vi "SQLite Adding Tests.vi"(8 "Error In (no error)":errorcluster) -> (0 "Error Out":errorcluster)   [LabVIEW 2023]
uses:
  <vilib>/addons/_JKI Toolkits/Caraya/classes/Test/Test.lvclass
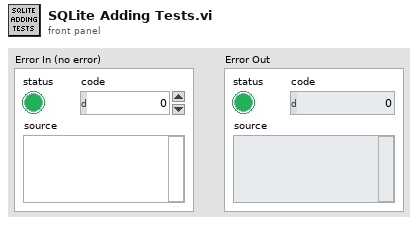
[diagram p1: front panel]
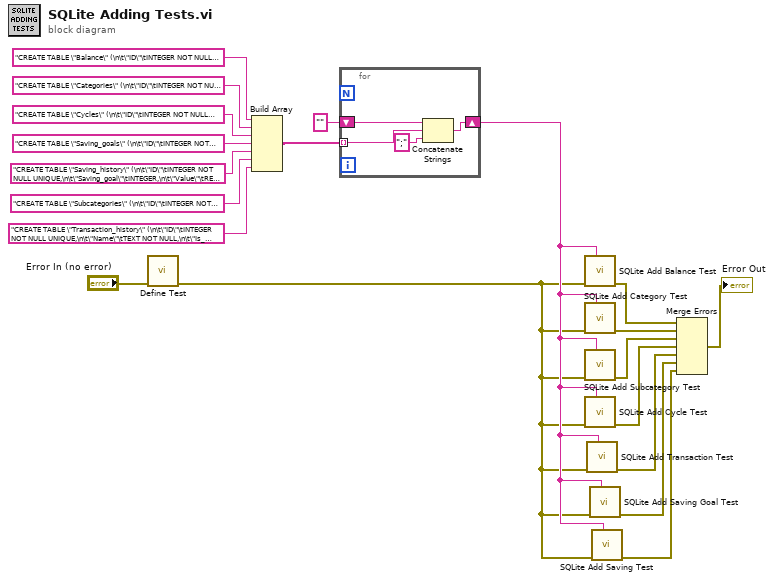
[diagram p0: block diagram]
diagram:
  n1 = call <vilib>:"Define Test.vi"("error in (no error)"="Error In (no error)") -> ("error out"=w2:errorcluster)  [unwired: 9 in, 1 out]
  n2 = Build Array("CREATE TABLE \"Balance\" (\n\t\"ID\"\tINTEGER NOT NULL UNIQUE,\n\t\"Value\"\tREAL NOT NULL,\n\t\"Last_update\"\tREAL NOT NULL,\n\tPRIMARY KEY(\"ID\" AUTOINCREMENT)\n);\nCREATE TRIGGER Balance_single AFTER INSERT ON Balance\nBEGIN\n  DELETE FROM Balance WHERE ID NOT IN (SELECT ID FROM Balance ORDER BY ID DESC LIMIT 1);\nEND", "CREATE TABLE \"Categories\" (\n\t\"ID\"\tINTEGER NOT NULL UNIQUE,\n\t\"Name\"\tTEXT NOT NULL UNIQUE,\n\tPRIMARY KEY(\"ID\" AUTOINCREMENT)\n)", "CREATE TABLE \"Cycles\" (\n\t\"ID\"\tINTEGER NOT NULL UNIQUE,\n\t\"Name\"\tTEXT NOT NULL UNIQUE,\n\t\"Day_of_occurence\"\tINTEGER NOT NULL CHECK(Day_of_occurence >= 1 AND Day_of_occurence <= 31),\n\t\"Description\"\tTEXT,\n\tPRIMARY KEY(\"ID\" AUTOINCREMENT)\n)", "CREATE TABLE \"Saving_goals\" (\n\t\"ID\"\tINTEGER NOT NULL UNIQUE,\n\t\"Name\"\tTEXT NOT NULL,\n\t\"Current_value\"\tREAL NOT NULL,\n\t\"Target_value\"\tREAL NOT NULL CHECK(\"Target_value\" >= 0),\n\t\"Date_of_entry\"\tREAL NOT NULL,\n\t\"Due_date\"\tREAL CHECK(\"Due_date\" IS NULL OR \"Due_date\" > \"Date_of_entry\"),\n\t\"Last_update\"\tREAL NOT NULL,\n\t\"Description\"\tTEXT,\n\tPRIMARY KEY(\"ID\" AUTOINCREMENT)\n)", "CREATE TABLE \"Saving_history\" (\n\t\"ID\"\tINTEGER NOT NULL UNIQUE,\n\t\"Saving_goal\"\tINTEGER,\n\t\"Value\"\tREAL NOT NULL,\n\t\"Date_of_entry\"\tREAL NOT NULL,\n\t\"Description\"\tTEXT,\n\tFOREIGN KEY(\"Saving_goal\") REFERENCES \"Saving_goals\"(\"ID\") ON DELETE SET NULL,\n\tPRIMARY KEY(\"ID\" AUTOINCREMENT)\n);\nCREATE TRIGGER SavingGoalInsert\nAFTER INSERT ON Saving_history\nBEGIN\n    UPDATE Saving_goals\n    SET Current_value = Current_value + NEW.Value\n    WHERE ID = New.Saving_goal;\nEND;\nCREATE TRIGGER SavingGoalUpdate\nAFTER UPDATE ON Saving_history\nBEGIN\n    UPDATE Saving_goals\n    SET Current_value = Current_value -OLD.Value+ NEW.Value\n    WHERE ID = New.Saving_goal;\nEND", "CREATE TABLE \"Subcategories\" (\n\t\"ID\"\tINTEGER NOT NULL UNIQUE,\n\t\"Name\"\tTEXT NOT NULL,\n\t\"Category\"\tINTEGER NOT NULL,\n\tFOREIGN KEY(\"Category\") REFERENCES \"Categories\"(\"ID\") ON DELETE CASCADE,\n\tPRIMARY KEY(\"ID\" AUTOINCREMENT)\n)", "CREATE TABLE \"Transaction_history\" (\n\t\"ID\"\tINTEGER NOT NULL UNIQUE,\n\t\"Name\"\tTEXT NOT NULL,\n\t\"Is_income\"\tINTEGER NOT NULL,\n\t\"Value\"\tREAL NOT NULL CHECK(NOT (\"Value\" = 0)),\n\t\"Amount\"\tREAL NOT NULL CHECK(NOT (\"Amount\" = 0)),\n\t\"Total\"\tREAL GENERATED ALWAYS AS (\"Amount\" * \"Value\") STORED,\n\t\"Date_of_entry\"\tREAL NOT NULL,\n\t\"Date_of_occurence\"\tREAL,\n\t\"Last_update\"\tREAL NOT NULL,\n\t\"Category\"\tINTEGER,\n\t\"Subcategory\"\tINTEGER,\n\t\"Cycle\"\tINTEGER,\n\t\"Description\"\tTEXT,\n\tFOREIGN KEY(\"Category\") REFERENCES \"Categories\"(\"ID\") ON DELETE SET NULL,\n\tFOREIGN KEY(\"Cycle\") REFERENCES \"Cycles\"(\"ID\") ON DELETE SET NULL,\n\tFOREIGN KEY(\"Subcategory\") REFERENCES \"Subcategories\"(\"ID\") ON DELETE SET NULL,\n\tPRIMARY KEY(\"ID\" AUTOINCREMENT)\n);CREATE TRIGGER ReplaceNullValue\nAFTER INSERT ON Transaction_history\nBEGIN\n    UPDATE Transaction_history\n    SET Date_of_occurence = COALESCE(Date_of_occurence, Date_of_entry)\n    WHERE ID = NEW.ID;\nEND") -> (w11:string[])
  n3 = for {
    tunnel: w11 -> [w24] mode=indexing
    shift-right: [w22] -> w3
    shift-left: "" -> [w21]
    n4 = Concatenate Strings(w21, w24, ";" ("string")) -> (w22:string)
  }
  n5 = call "SQLite Add Balance Test.vi"("Test DB Set Up Command"=w3, "Error In (no error)"=w2) -> ("Error Out"=w9:errorcluster)  [unwired: 8 in, 1 out]
  n6 = call "SQLite Add Category Test.vi"("Test DB Set Up Command"=w3, "Error In (no error)"=w2) -> ("Error Out"=w10:errorcluster)  [unwired: 8 in, 1 out]
  n7 = call "SQLite Add Subcategory Test.vi"("Test DB Set Up Command"=w3, "Error In (no error)"=w2) -> ("Error Out"=w8:errorcluster)  [unwired: 8 in, 1 out]
  n8 = call "SQLite Add Cycle Test.vi"("Test DB Set Up Command"=w3, "Error In (no error)"=w2) -> ("Error Out"=w6:errorcluster)  [unwired: 8 in, 1 out]
  n9 = call "SQLite Add Transaction Test.vi"("Test DB Set Up Command"=w3, "Error In (no error)"=w2) -> ("Error Out"=w5:errorcluster)  [unwired: 8 in, 1 out]
  n10 = call "SQLite Add Saving Goal Test.vi"("Test DB Set Up Command"=w3, "Error In (no error)"=w2) -> ("Error Out"=w4:errorcluster)  [unwired: 8 in, 1 out]
  n11 = call "SQLite Add Saving Test.vi"("Test DB Set Up Command"=w3, "Error In (no error)"=w2) -> ("Error Out"=w1:errorcluster)  [unwired: 8 in, 1 out]
  n12 = Merge Errors(w9, w10, w8, w6, w5, w4, w1) -> (→"Error Out":errorcluster)
